vi "ResizeToBiggestDecoration.vi"(8 "error in (no error)":errorcluster, 11 "VI in":refnum<vi>) -> (0 "error out":errorcluster)   [LabVIEW 2022 SP3]
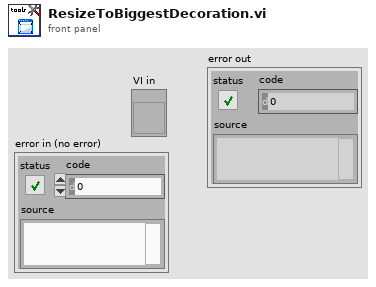
[diagram p1: front panel]
types:
  T1 = typedef "LVBoundsTypeDef.ctl" = cluster{"Width":u32, "Height":u32}
  T2 = typedef "LVPositionTypeDef.ctl" = cluster{"Left":i32, "Top":i32}
  T3 = typedef "LVRectTypeDef.ctl" = cluster{"Left":i16, "Top":i16, "Right":i16, "Bottom":i16}
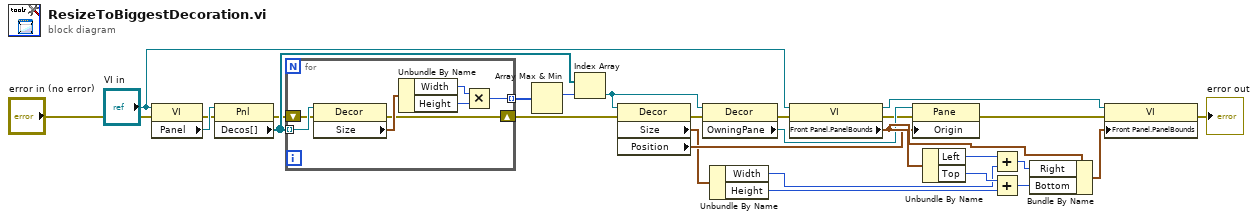
[diagram p0: block diagram]
diagram:
  n1 = property class="VI"(reference="VI in", error in="error in (no error)") -> (error out=w9:errorcluster, "Panel"=w13:refnum<vi>)  [unwired: 1 out]
  n2 = property class="Pnl"(reference=w13, error in=w9) -> (error out=w8:errorcluster, "Decos[]"=w12:refnum<vi>[])  [unwired: 1 out]
  n3 = for {
    tunnel: w12 -> [w34] mode=indexing
    tunnel: [w30] -> w10 mode=indexing
    shift-right: [w28] -> w7
    shift-left: w8 -> [w29]
    n4 = property class="Decor"(reference=w34, error in=w29) -> (error out=w28:errorcluster, "Size"=w33:T1)  [unwired: 1 out]
    n5 = Unbundle By Name(w33) -> ("Width"=w31:u32, "Height"=w32:u32)
    n6 = Multiply(x=w31, y=w32) -> (x*y=w30:u32)
  }
  n7 = Array Max & Min(array=w10) -> (max index (indices)=w11:i32)  [unwired: 3 out]
  n8 = Index Array(array=w12, index=w11) -> (element=w19:refnum<vi>)
  n9 = property class="Decor"(reference=w19, error in=w7) -> (error out=w6:errorcluster, "Size"=w14:T1, "Position"=w21:T2)  [unwired: 1 out]
  n10 = property class="Decor"(reference=w19, error in=w6) -> (error out=w5:errorcluster, "OwningPane"=w20:refnum<vi>)  [unwired: 1 out]
  n11 = Unbundle By Name(w14) -> ("Width"=w15:u32, "Height"=w17:u32)
  n12 = property class="VI"(reference="VI in", error in=w5) -> (reference out=w23:refnum<vi>, error out=w4:errorcluster, "Front Panel.PanelBounds"=w26:T3)
  n13 = property class="Pane"(reference=w20, error in=w4, "Origin"=w21) -> (error out=w3:errorcluster)  [unwired: 1 out]
  n14 = Unbundle By Name(w26) -> ("Left"=w24:i16, "Top"=w27:i16)
  n15 = Add(x=w24, y=w15) -> (x+y=w16:u32)
  n16 = Add(x=w27, y=w17) -> (x+y=w18:u32)
  n17 = Bundle By Name(cluster=w26, "Right"=w16, "Bottom"=w18) -> (w25:T3)
  n18 = property class="VI"(reference=w23, error in=w3, "Front Panel.PanelBounds"=w25) -> (error out=→"error out":errorcluster)  [unwired: 1 out]
